vi "VideoLan.vi"() -> ()   [LabVIEW 2011]
uses:
  <instrlib>/niHWS/nihws.llb/niHWS Open File Permissions ID.ctl
  <instrlib>/niHWS/nihws.llb/niHWS Write Analog DBL.vi
panel:
  in  "Magnify":bool
  in  "stop":bool
  out "Camera":T1(plugin-control)
  out "Rec Time":dbl format="%#_3g"
  out "fps":dbl format="%#_2g"
  in  "Rec":bool
  in  "Path":path
  in  "Gain":dbl(slide)=2.6607250597988097 min=1.0 max=3.9810717055349722 scale=0.0..4.0
  in  "Exposure Time":dbl(slide)=16602.0 min=56.0 max=16602.0 scale=0.0..16600.0
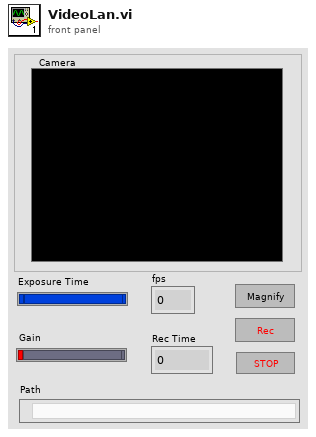
[diagram p1: front panel]
types:
  T1 = typedef "IMAQ Image.ctl" = refnum<image>
  T2 = enum32{"Invalid", "Standard", "Closed", "Hidden", "Minimized", "Maximized"}
  T3 = typedef "niHWS Open File Permissions ID.ctl" = enum32{"Read Only", "Read/Write Existing", "Read/Write/Create New", "Read/Write/Create New Always"}
  T4 = typedef "AviRefnum.ctl" = refnum<k1>
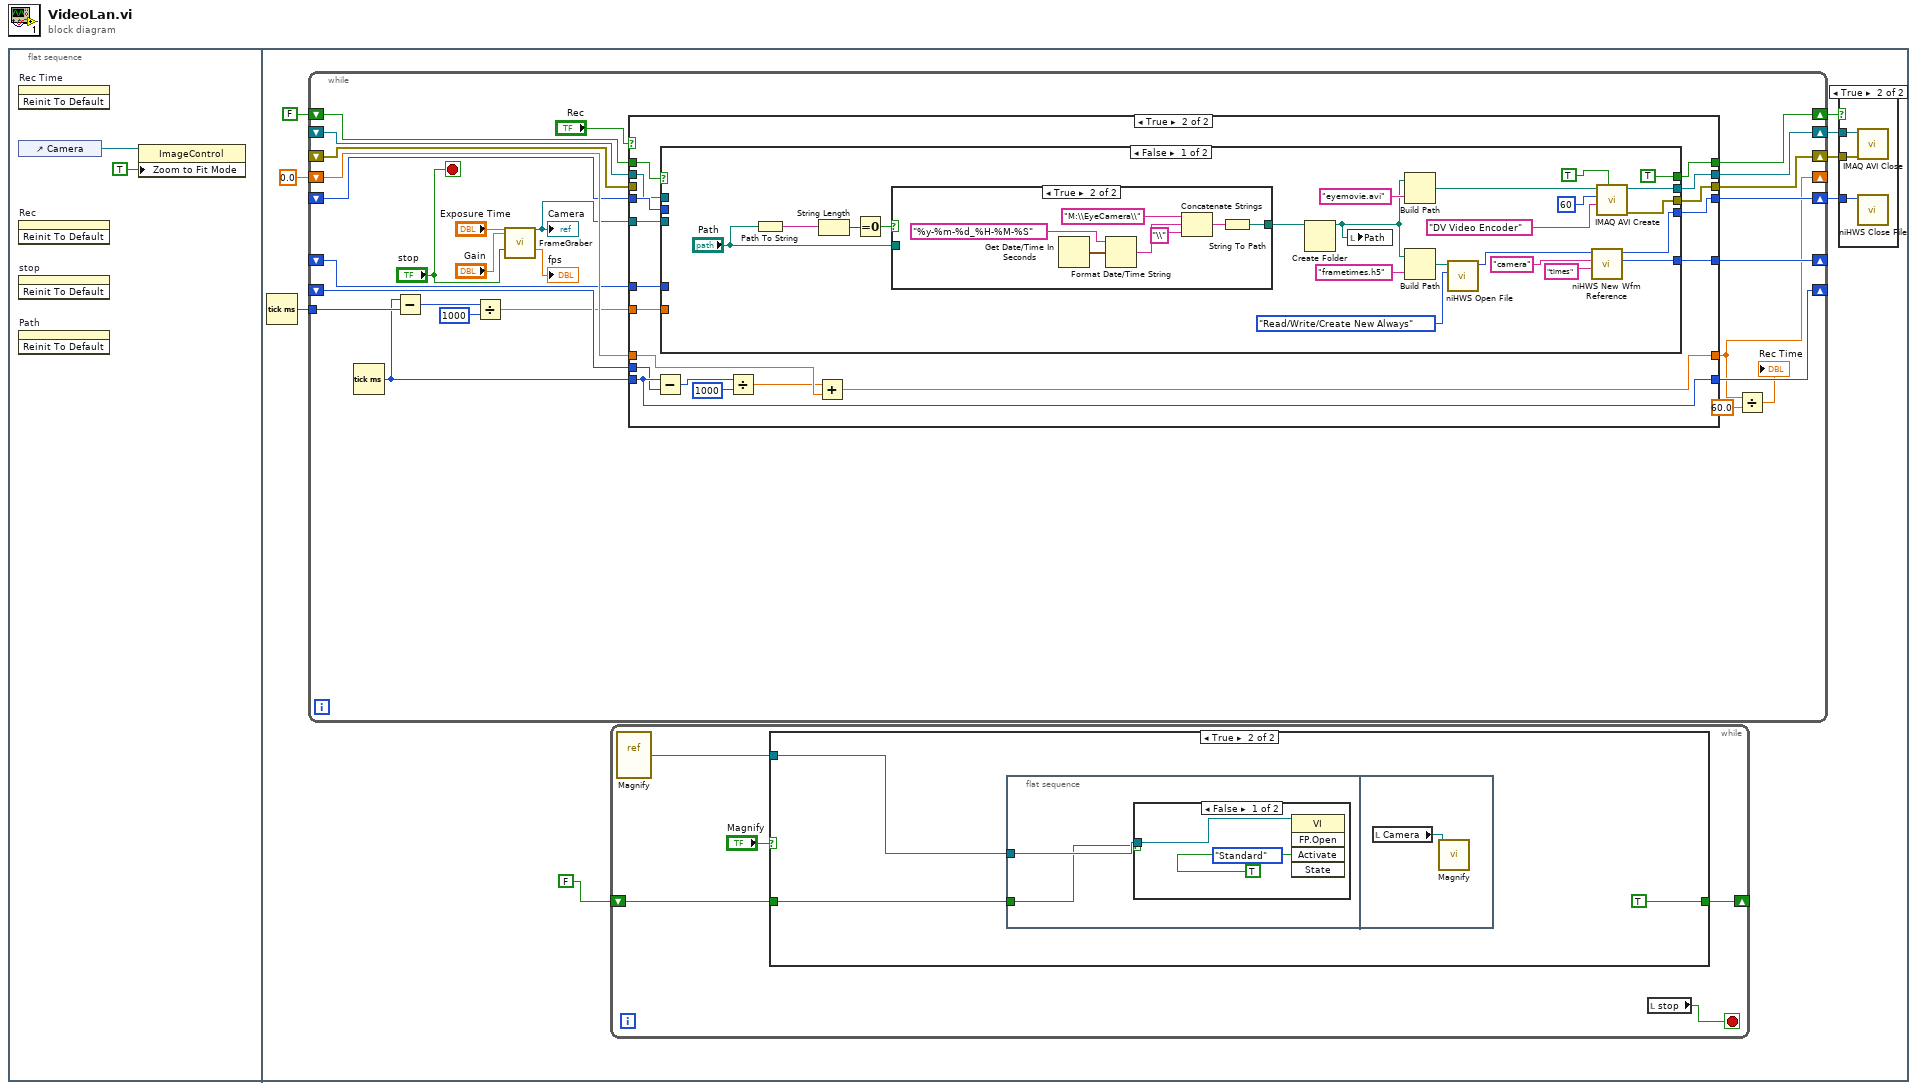
[diagram p0: block diagram]
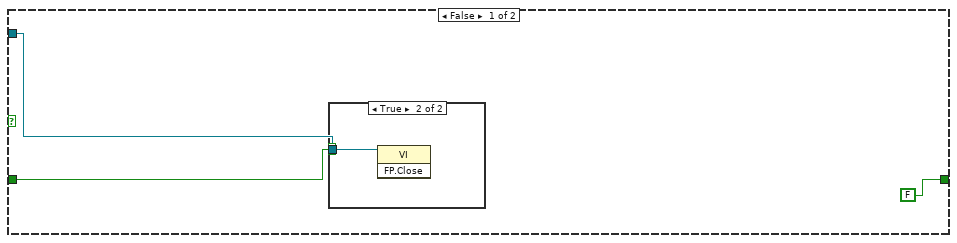
[diagram p2: hidden frame]
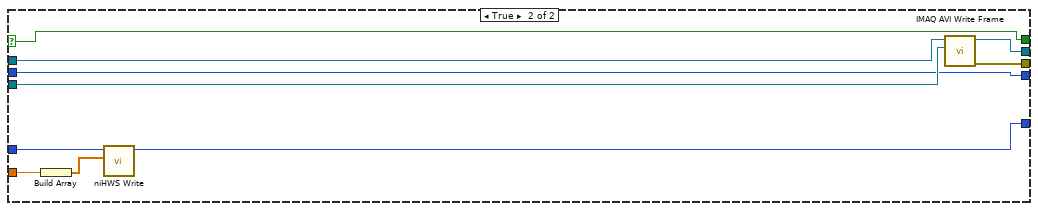
[diagram p8: hidden frame]
diagram:
  n1 = flat-sequence {
    frame #0 {
      n2 = invoke on="Rec Time" class="DigNum (strict)" method="Reinit To Default"() -> ()  [unwired: 3 in, 3 out]
      n3 = control-ref of="Camera"() -> (w2:refnum<vi>)
      n4 = invoke on="Rec" class="Bool (strict)" method="Reinit To Default"() -> ()  [unwired: 3 in, 3 out]
      n5 = invoke on="stop" class="Bool (strict)" method="Reinit To Default"() -> ()  [unwired: 3 in, 3 out]
      n6 = invoke on="Path" class="Path" method="Reinit To Default"() -> ()  [unwired: 3 in, 3 out]
      n7 = property on="Property Node" class="ImageControl"(reference=w2, "Zoom to Fit Mode"=TRUE) -> ()  [unwired: 1 in, 2 out]
    }
    frame #1 {
      n8 = Tick Count (ms)() -> (millisecond timer value=w7:u32)
      n9 = while {
        tunnel: w7 -> [w56]
        shift-right: [w55] -> _
        shift-left: _ -> [w54]
        shift-right: [w34] -> _
        shift-left: 0.0 -> [w53]
        shift-right: [w43] -> w5
        shift-left: FALSE -> [w44]
        shift-right: [w40] -> _
        shift-left: _ -> [w39]
        shift-right: [w41] -> w4
        shift-left: _ -> [w38]
        shift-right: [w58] -> w10
        shift-left: _ -> [w37]
        shift-right: [w57] -> w9
        shift-left: _ -> [w36]
        stop <- "stop" stop-if-true
        n10 = Tick Count (ms)() -> (millisecond timer value=w45:u32)
        n11 = Subtract(x=w45, y=w56) -> (x-y=w48:u32)
        n12 = Divide(x=w48, y=1000) -> (x/y=w46:dbl)
        n13 = call "FrameGraber.vi"("Exposure Time"="Exposure Time", "Gain"="Gain", "Stop (F)"="stop") -> ("Image Out"=w35:T1, "Frame Rate"=→"fps":dbl)  [unwired: 20 in, 3 out]
        "Camera" <- w35
        n14 = case shown="True" "Rec" {
          tunnel: [w60 w74] -> w58
          tunnel: [w59 w73] -> w57
          tunnel: [w64 w80] -> w34
          tunnel: w46 -> [_ w71]
          tunnel: [w65 w83] -> w55
          tunnel: w45 -> [w65 w83]
          tunnel: w54 -> [_ w82]
          tunnel: w53 -> [w64 w81]
          tunnel: w35 -> [_ w72]
          tunnel: w44 -> [w63 w76]
          tunnel: [w63 w75] -> w43
          tunnel: [w61 w70] -> w41
          tunnel: [w62 w69] -> w40
          tunnel: w39 -> [w62 w68]
          tunnel: w38 -> [w61 w67]
          tunnel: w37 -> [w60 w66]
          tunnel: w36 -> [w59 _]
          frame False {
          }
          frame True {
            n15 = Subtract(x=w83, y=w82) -> (x-y=w79:u32)
            n16 = case shown="False" w76 {
              selector: w76 -> [_ w123]
              tunnel: [TRUE w123] -> w75
              tunnel: [w102 w122] -> w74
              tunnel: [w101 w121] -> w73
              tunnel: w72 -> [_ w120]
              tunnel: w71 -> [_ w118]
              tunnel: [w88 w115] -> w70
              tunnel: [w87 w116] -> w69
              tunnel: w68 -> [_ w117]
              tunnel: w67 -> [_ w115]
              tunnel: w66 -> [_ w114]
              frame False {
                n17 = Path To String(path="Path") -> (string=w103:string)
                n18 = String Length(string=w103) -> (length=w104:i32)
                n19 = Equal To 0?(x=w104) -> (x = 0?=w89:bool)
                n20 = case shown="True" w89 {
                  tunnel: [w106 w107] -> w85
                  tunnel: "Path" -> [w106 _]
                  frame False {
                  }
                  frame True {
                    n21 = Get Date/Time In Seconds() -> (seconds since 1Jan1904=w113:timestamp)
                    n22 = Format Date/Time String(time format string (%c)="%y-%m-%d_%H-%M-%S", seconds (now)=w113) -> (date/time string=w110:string)  [unwired: 1 in]
                    n23 = Concatenate Strings("M:\\EyeCamera\\", w110, "\\" ("string")) -> (w108:string)
                    n24 = String To Path(string=w108) -> (path=w107:path)
                  }
                }
                n25 = Create Folder(path (use dialog)=w85) -> (created path=w84:path)  [unwired: 2 in, 2 out]
                n26 = local write "Path"(w84) -> ()
                n27 = Build Path(base path=w84, name or relative path="eyemovie.avi" ("search string")) -> (appended path=w95:path)
                n28 = Build Path(base path=w84, name or relative path="frametimes.h5" ("search string")) -> (appended path=w90:path)
                n29 = call <instrlib>:"niHWS Open File.vi"("permissions (0:read only)"=niHWS_Open_File_Permissions_ID."Read/Write/Create New Always", "file path"=w90) -> ("file handle"=w94:u32)  [unwired: 8 in, 1 out]
                n30 = call <instrlib>:"niHWS New Wfm Reference.vi"("waveform name (empty)"="times" ("group name (empty)"), "group name (empty)"="camera", "file handle in"=w94) -> ("waveform reference"=w87:u32, "file handle out"=w88:u32)  [unwired: 6 in, 1 out]
                n31 = call "IMAQ AVI Create"("Has Data"=TRUE, "Compression Filter"="DV Video Encoder" ("Compressor"), "Frames Per Second"=u32 60, "AVI Path"=w95) -> ("error out"=w101:errorcluster, "Avi Refnum"=w102:T4)  [unwired: 3 in, 3 out]
              }
              frame True {
                n32 = Build Array(w118) -> (w119:dbl[])
                n33 = call-poly <instrlib>:"niHWS Write.vi"("data"=w119, "waveform reference in"=w117) -> ("waveform reference out"=w116:u32)  [unwired: 8 in, 1 out]
                n34 = call "IMAQ AVI Write Frame"("Image"=w120, "Avi Refnum"=w114) -> ("error out"=w121:errorcluster, "Avi Refnum (duplicate)"=w122:T4)  [unwired: 8 in]
              }
            }
            n35 = Divide(x=w79, y=1000) -> (x/y=w77:dbl)
            n36 = Add(x=w77, y=w81) -> (x+y=w80:dbl)
          }
        }
        n37 = Divide(x=w34, y=60.0) -> (x/y=→"Rec Time":dbl)
      }
      n38 = while {
        shift-right: [w12] -> _
        shift-left: FALSE -> [w11]
        stop <- w13 stop-if-true
        n39 = vi-ref "Magnify.vi"() -> (w15:refnum<vi>)
        n40 = case shown="True" "Magnify" {
          tunnel: w15 -> [w18 w22]
          tunnel: [FALSE TRUE] -> w12
          tunnel: w11 -> [w17 w20]
          frame False {
            n41 = case shown="True" w17 {
              tunnel: w18 -> [_ w19]
              frame False {
              }
              frame True {
                n42 = invoke class="VI" method="FP.Close"(reference=w19) -> ()  [unwired: 2 in, 3 out]
              }
            }
          }
          frame True {
            n43 = flat-sequence {
              tunnel: w22 -> [w24]
              tunnel: w20 -> [w23]
              frame #0 {
                n44 = case shown="False" w23 {
                  tunnel: w24 -> [w26 _]
                  frame False {
                    n45 = invoke class="VI" method="FP.Open"(reference=w26, "Activate"=TRUE ("Wait Until Done"), "State"=T2."Standard") -> ()  [unwired: 2 in, 5 out]
                  }
                  frame True {
                  }
                }
              }
              frame #1 {
                n46 = local read "Camera"() -> (w28:T1)
                n47 = call "Magnify.vi"("Camera 2"=w28) -> ()  [unwired: 11 in]
              }
            }
          }
        }
        n48 = local read "stop"() -> (w13:bool)
      }
      n49 = case shown="True" w5 {
        tunnel: w10 -> [_ w31]
        tunnel: w9 -> [_ w30]
        tunnel: w4 -> [_ w29]
        frame False {
        }
        frame True {
          n50 = call "IMAQ AVI Close"("error in (no error)"=w30, "Avi Refnum"=w31) -> ()  [unwired: 9 in, 1 out]
          n51 = call <instrlib>:"niHWS Close File.vi"("file handle"=w29) -> ()  [unwired: 10 in, 1 out]
        }
      }
    }
  }
